vi "algo.shift.not.final.vi"(11 "algo.data.in":T1={"next.state"=enum."Noop", "saved.state"=enum."Noop", "scratch"={"i"=0, "n"=0, "start.addr"=0, "first.call?"=FALSE, "j"=0, "o"=0, "k"=0, "p"=0, "just.write"=FALSE, "orderId "=0, "dir"=0}, "mode"=enum."Get.Symbol", "cmd.mem.watchlist"={"read.request"=FALSE, "read.addr"=0, "read.ready"=FALSE, "val.watchlist.read"={"symbol"=0, "buy.start.addr"=0, "buy.size"=0, "buy.slots"=0, "sell.start.addr"=0, "sell.size"=0, "sell.slots"=0, "min.ask"=0, "max.bid"=0}, "write.request"=FALSE, "write.addr"=0, "val.watchlist.write"={"symbol"=0, "buy.start.addr"=0, "buy.size"=0, "buy.slots"=0, "sell.start.addr"=0, "sell.size"=0, "sell.slots"=0, "min.ask"=0, "max.bid"=0}}, "cmd.mem.orders"={"read.addr"=0, "read.request"=FALSE, "read.ready"=FALSE, "write.addr"=0, "write.request"=FALSE, "read.data"={"OrderId"=0, "Price"=0, "Quantity"=0}, "write.data"={"OrderId"=0, "Price"=0, "Quantity"=0}}, "cmd.state"={"write.to.state"=FALSE, "val.state"=[0, 0, 0, 0]}, "cmd.debug"={"write.to.debug"=FALSE, "val.debug"=[0, 0]}, "stats"={"min.ask"=0, "max.bid"=0, "price"=0, "quantity"=0, "execution"=FALSE}, "orderbook.command"={"type"=enum."Time", "side"=0, "orderId "=0, "quantity"=0, "symbol"=0, "price"=0, "executed.qty"=0, "canceled.qty"=0, "remaining.qty"=0, "seconds"=0, "nanoseconds"=0, "Add"=FALSE, "Edit"=FALSE, "Remove"=FALSE}, "time"={"last"=0, "since"=0}, "watchlist.size"=0, "active.watchlist"={"item"={"symbol"=0, "buy.start.addr"=0, "buy.size"=0, "buy.slots"=0, "sell.start.addr"=0, "sell.size"=0, "sell.slots"=0, "min.ask"=0, "max.bid"=0}, "index"=0}, "active.order"={"buy"=FALSE, "sell"=FALSE, "addr"=0, "size"=0, "slots"=0, "index"=0}} {"active.watchlist"."item"."symbol" format="%.0x"; "cmd.mem.orders"."write.data"."OrderId" format="%.0x"; "cmd.mem.orders"."read.data"."OrderId" format="%.0x"; "cmd.mem.watchlist"."val.watchlist.write"."symbol" format="%.0x"; "cmd.mem.watchlist"."val.watchlist.read"."symbol" format="%.0x"}) -> (2 "dbg.val.1":u64, 3 "write_ob.cmd":bool)   [LabVIEW 2022 SP3]
uses:
  algo.data.ctl
  types/algo.states.ctl
  types/algo.scratch.ctl
  types/algo.mode.ctl
  types/algo.cmd.mem.watchlist.ctl
  types/algo.val.watchlist.ctl
  types/algo.cmd.mem.orders.ctl
  types/algo.val.order.ctl
  types/algo.cmd.state.ctl
  types/algo.val.state.ctl
  types/algo.cmd.debug.ctl
  types/algo.val.debug.ctl
  types/algo.stats.ctl
  common/orderbook.command.ctl
  common/orderbook.command.type.ctl
  types/algo.time.ctl
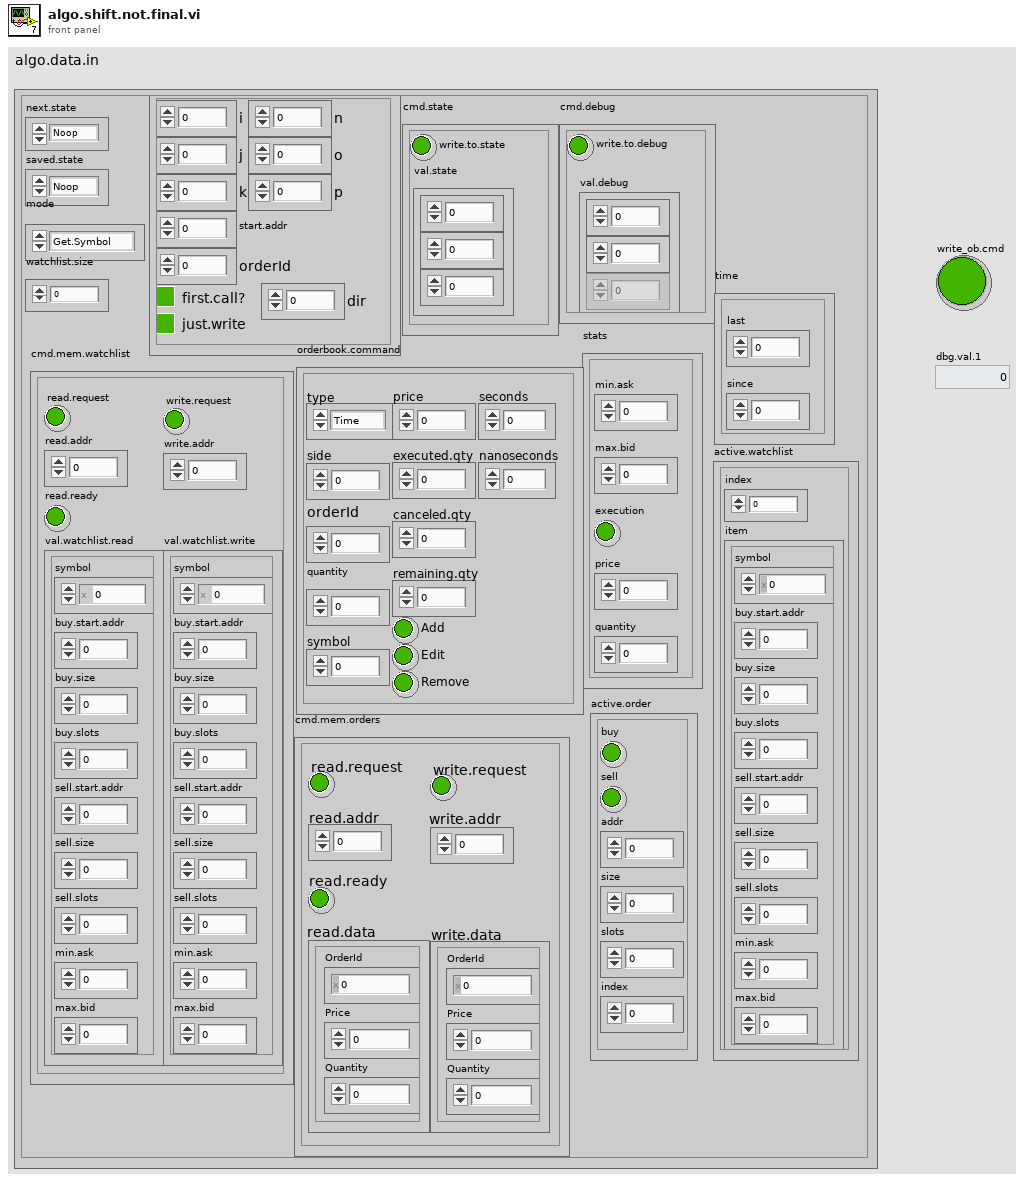
[diagram p1: front panel]
types:
  T1 = typedef "algo.data.ctl" = cluster{"next.state":T2, "saved.state":T2, "scratch":T3, "mode":T4, "cmd.mem.watchlist":T5, "cmd.mem.orders":T7, "cmd.state":T9, "cmd.debug":T11, "stats":T13, "orderbook.command":T14, "time":T16, "watchlist.size":u64, "active.watchlist":cluster{"item":T6, "index":u64}, "active.order":cluster{"buy":bool, "sell":bool, "addr":i16, "size":i16, "slots":i16, "index":i16}}
  T2 = typedef "algo.states.ctl" = enum16{"Noop", "Reset", "Configuration", "Debug", "Get.State", "Wait.for.Command", "Process.Command"}
  T3 = typedef "algo.scratch.ctl" = cluster{"i":u64, "n":u64, "start.addr":u16, "first.call?":bool, "j":u64, "o":u64, "k":u64, "p":u64, "just.write":bool, "orderId ":u64, "dir":i8}
  T4 = typedef "algo.mode.ctl" = enum16{"watchlist.iter", "order.buy.iter", "order.sell.iter", "Get.Symbol", "Search", "Shift"}
  T5 = typedef "algo.cmd.mem.watchlist.ctl" = cluster{"read.request":bool, "read.addr":u16, "read.ready":bool, "val.watchlist.read":T6, "write.request":bool, "write.addr":u16, "val.watchlist.write":T6}
  T6 = typedef "algo.val.watchlist.ctl" = cluster{"symbol":u64, "buy.start.addr":u16, "buy.size":u16, "buy.slots":u16, "sell.start.addr":u16, "sell.size":u16, "sell.slots":u16, "min.ask":u64, "max.bid":u64}
  T7 = typedef "algo.cmd.mem.orders.ctl" = cluster{"read.addr":u16, "read.request":bool, "read.ready":bool, "write.addr":u16, "write.request":bool, "read.data":T8, "write.data":T8}
  T8 = typedef "algo.val.order.ctl" = cluster{"OrderId":u64, "Price":u64, "Quantity":u32}
  T9 = typedef "algo.cmd.state.ctl" = cluster{"write.to.state":bool, "val.state":T10}
  T10 = typedef "algo.val.state.ctl" = u64[]
  T11 = typedef "algo.cmd.debug.ctl" = cluster{"write.to.debug":bool, "val.debug":T12}
  T12 = typedef "algo.val.debug.ctl" = u64[]
  T13 = typedef "algo.stats.ctl" = cluster{"min.ask":u32, "max.bid":u32, "price":u32, "quantity":u32, "execution":bool}
  T14 = typedef "orderbook.command.ctl" = cluster{"type":T15, "side":u8, "orderId ":u64, "quantity":u32, "symbol":u64, "price":u64, "executed.qty":u32, "canceled.qty":u32, "remaining.qty":u32, "seconds":u64, "nanoseconds":u64, "Add":bool, "Edit":bool, "Remove":bool}
  T15 = typedef "orderbook.command.type.ctl" = enum8{"Time", "AddOrder", "OrderExecuted", "OrderExecutedAtPrice", "ReduceSize", "ModifyOrder", "DeleteOrder", "Get.Everything", "Get.All.Orders", "Get.Top"}
  T16 = typedef "algo.time.ctl" = cluster{"last":u32, "since":u32}
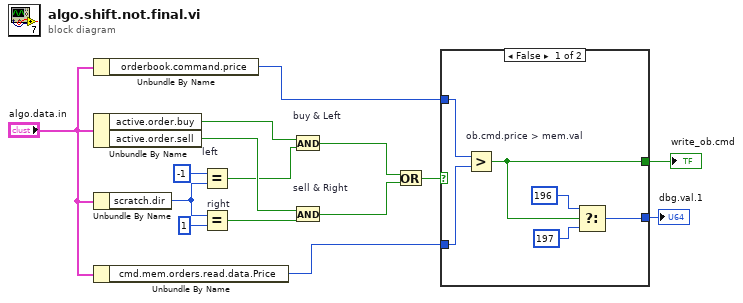
[diagram p0: block diagram]
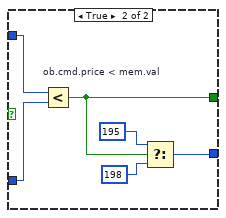
[diagram p2: hidden frame]
diagram:
  n1 = Unbundle By Name("algo.data.in") -> ("orderbook.command.price"=w10:u64)
  n2 = Unbundle By Name("algo.data.in") -> ("active.order.buy"=w15:bool, "active.order.sell"=w14:bool)
  n3 = Unbundle By Name("algo.data.in") -> ("scratch.dir"=w5:i8)
  n4 = Unbundle By Name("algo.data.in") -> ("cmd.mem.orders.read.data.Price"=w9:u64)
  n5 = Equal? "left"(x=i8 -1, y=w5) -> (x = y?=w3:bool)
  n6 = Equal? "right"(x=w5, y=i8 1) -> (x = y?=w4:bool)
  n7 = And "buy & Left"(x=w15, y=w3) -> (x .and. y?=w13:bool)
  n8 = And "sell & Right"(x=w14, y=w4) -> (x .and. y?=w12:bool)
  n9 = Or(x=w13, y=w12) -> (x .or. y?=w11:bool)
  n10 = case shown="False" w11 {
    tunnel: w10 -> [w21 w27]
    tunnel: w9 -> [w20 w26]
    tunnel: [w16 w24] -> w8
    tunnel: [w17 w25] -> w7
    frame False {
      n11 = Greater? "ob.cmd.price > mem.val"(x=w21, y=w20) -> (0:w16:bool)
      n12 = Select(t=u64 196 ("dbg.val.1"), s=w16, f=u64 197 ("dbg.val.1")) -> (s? t:f=w17:u64)
    }
    frame True {
      n13 = Less? "ob.cmd.price < mem.val"(x=w27, y=w26) -> (x < y?=w24:bool)
      n14 = Select(t=u64 195 ("dbg.val.1"), s=w24, f=u64 198 ("dbg.val.1")) -> (s? t:f=w25:u64)
    }
  }
  "write_ob.cmd" <- w8
  "dbg.val.1" <- w7
